vi "HatchModeToDash.vi"(10 "Update?":bool, 11 "HatchModeIn":T1) -> (3 "HatchModeOut":T1)   [LabVIEW 2018]
uses:
  HatchModes.ctl
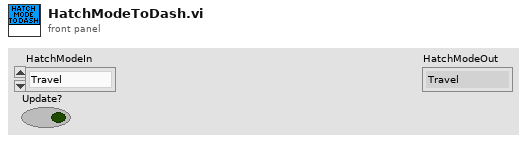
[diagram p1: front panel]
types:
  T1 = typedef "HatchModes.ctl" = enum16{"Travel", "PickPlace"}
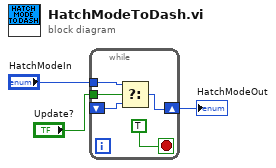
[diagram p0: block diagram]
diagram:
  n1 = while {
    tunnel: "Update?" -> [w8]
    tunnel: "HatchModeIn" -> [w7]
    shift-right: [w6] -> w1
    shift-left: _ -> [w5]
    stop <- TRUE stop-if-true
    n2 = Select(t=w7, s=w8, f=w5) -> (s? t:f=w6:T1)
  }
  "HatchModeOut" <- w1
